vi "From JSON.vi"(8 "error in (no error)":errorcluster, 10 "Path":path, 11 "DC Config in":refnum<class "DC Config.lvclass">) -> (0 "error out":errorcluster, 3 "DC Config out":refnum<class "DC Config.lvclass">)   [LabVIEW 2023, in "PXI-5441.lvlib" / "DC Config.lvclass"]
uses:
  DC Config.lvclass
  Signal Export Cluster.ctl
  <instrlib>/niFgen/niFgen.llb/niFgen_ctl Exported Signal Desination Values (ComboBox).ctl
  <instrlib>/niFgen/niFgen.llb/niFgen_ctl Exported Signal Name Values (Ring).ctl
  DC Config.lvclass/DC Config.ctl
  JSON/Set Cluster Values from JSON String.vi
  JSON/JSON.lvlib
panel:
  out "Settings Cluster":T4 {"Signal Export Cluster"."Signal to Export" items=["Sample Clock"=101, "Sample Clock Timebase"=1006, "Reference Clock"=102, "Onboard Reference Clock"=1019, "Start Trigger"=1004, "Script Trigger"=103, "Marker Event"=1001, "Data Marker Event"=108, "Ready For Start Event"=105, "Started Event"=106, "Done Event"=107, "Synchronization Pulse"=1007, "Sync Out"=1002]}
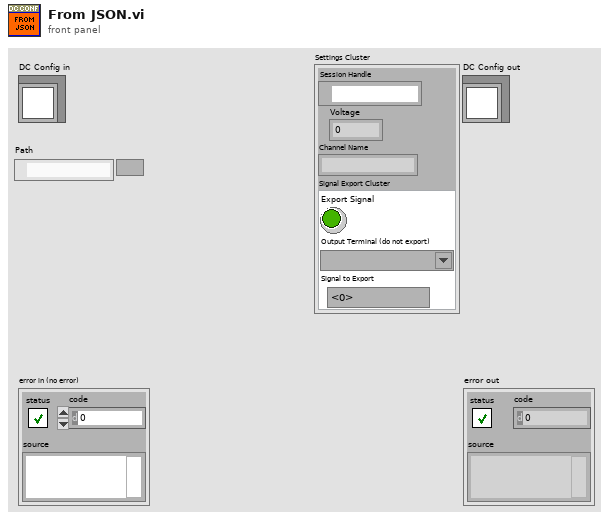
[diagram p1: front panel]
types:
  T1 = typedef "Signal Export Cluster.ctl" = cluster{"Export Signal":bool, "Output Terminal (do not export)":T2, "Signal to Export":T3}
  T2 = typedef "niFgen_ctl Exported Signal Desination Values (ComboBox).ctl" = string
  T3 = typedef "niFgen_ctl Exported Signal Name Values (Ring).ctl" = u16
  T4 = cluster{"Session Handle":refnum<k15>, "Voltage":dbl, "Channel Name":string, "Signal Export Cluster":T1}
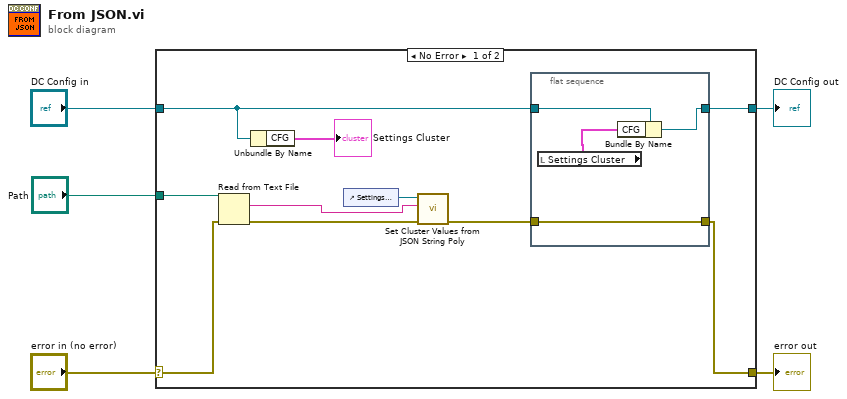
[diagram p0: block diagram]
diagram:
  n1 = case shown="No Error" "error in (no error)" {
    selector: "error in (no error)" -> [w12 w21]
    tunnel: [w8 w21] -> w4
    tunnel: [w6 w20] -> w2
    tunnel: "DC Config in" -> [w7 w20]
    tunnel: "Path" -> [w13 _]
    frame No Error {
      n2 = Read from Text File(file (use dialog)=w13, error in=w12) -> (text=w11:string, error out=w10:errorcluster)  [unwired: 2 in, 2 out]
      n3 = Unbundle By Name(w7) -> ("CFG"=→"Settings Cluster":T4)
      n4 = control-ref of="Settings Cluster"() -> (w14:refnum<vi>)
      n5 = call-poly "Set Cluster Values from JSON String Poly.vi"("error in (no error)"=w10, "JSON string"=w11, "Clust Refnum"=w14) -> ("error out"=w9:errorcluster)  [unwired: 8 in]
      n6 = flat-sequence {
        tunnel: w9 -> [w19]
        tunnel: [w19] -> w8
        tunnel: w7 -> [w18]
        tunnel: [w17] -> w6
        frame #0 {
          n7 = local read "Settings Cluster"() -> (w16:T4)
          n8 = Bundle By Name(cluster=w18, "CFG"=w16) -> (w17:refnum<class "DC Config.lvclass">)
        }
      }
    }
    frame Error {
    }
  }
  "error out" <- w4
  "DC Config out" <- w2
